vi "TSPopup.FG.Popup.vi"(4 "Popup Accepted?":bool, 6 "Popup Cluster Ref":refnum<vi>, 7 "Popup Operation":T5, 8 "error in (no error)":errorcluster, 9 "Font Size":u32, 10 "Encoded Location":string, 11 "Popup Parameters":T1) -> (0 "error out":errorcluster, 1 "Found":bool, 2 "Popup Parameters out":T1, 3 "Popup Event":refnum<user-event>)   [LabVIEW 2013]
doc: "The functional global that provides most of the functionality under the hood. This VI is wrapped by different public functions to provide a more user-friendly interface to the Type Sensitive Popup functions.\n\nType Sensitive Popup \nCopyright © 2007, J. David Saunders\nAll rights reserved."
uses:
  TSPopup.Popup Results.ctl
  TSPopup.Popup Operation.ctl
  TSPopup.Popup Call Parameters.ctl
  TSPopup.Data Type.ctl
  TSPopup.Monitor Register Data.ctl
  TSPopup.Event Enum.ctl
panel:
  in  "Reg. Data (type only)":T3
  in  "Popup Results (type only)":T6
  # "Type Sensitive Popup \nCopyright © 2007, J. David Saunders\nAll rights reserved."
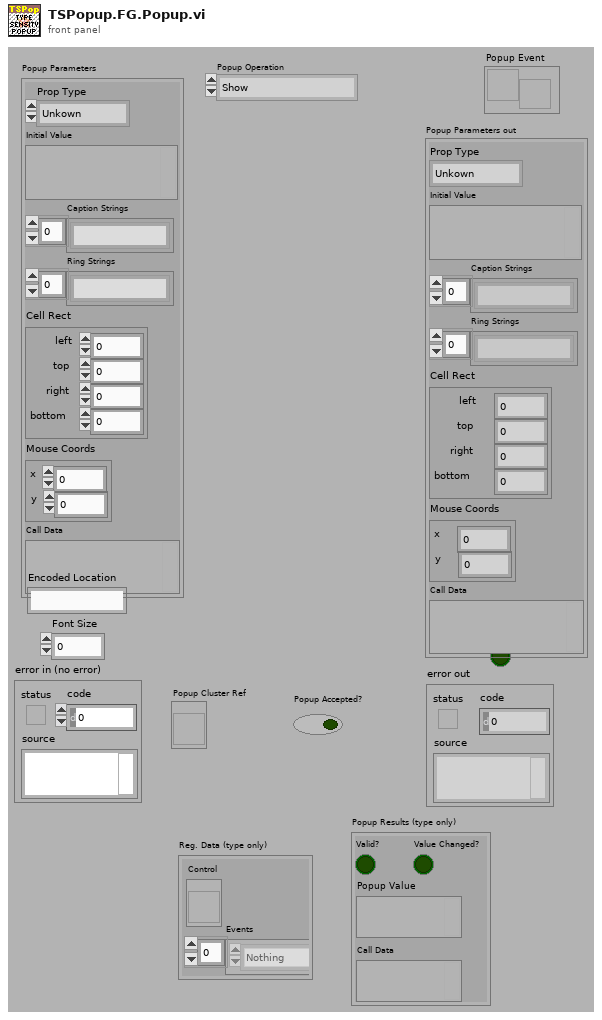
[diagram p1: front panel]
types:
  T1 = typedef "TSPopup.Popup Call Parameters.ctl" = cluster{"Prop Type":T2, "Initial Value":variant, "Caption Strings":string[], "Ring Strings":string[], "Cell Rect":cluster{"left":i16, "top":i16, "right":i16, "bottom":i16}, "Mouse Coords":cluster{"x":i16, "y":i16}, "Call Data":variant}
  T2 = typedef "TSPopup.Data Type.ctl" = enum16{"Unkown", "NO POPUP", "String", "Integer", "Float", "Color", "Boolean", "Ring", "Captioned String", "Captioned Integer", "Button Color", "2 Int Cluster", "4 Int Cluster"}
  T3 = typedef "TSPopup.Monitor Register Data.ctl" = cluster{"Control":refnum<vi>, "Events":T4[]}
  T4 = typedef "TSPopup.Event Enum.ctl" = enum16{"Nothing", "Enter Key Accept", "Escape Key Cancel", "Mouse Outside Accept", "Mouse Outside Cancel", "Mouse Move Accept", "Mouse Move Cancel", "Mouse Leave Cancel", "Value Change Accept", "Lose Focus Cancel", "Cancel Button", "Accept Button"}
  T5 = typedef "TSPopup.Popup Operation.ctl" = enum16{"Show", "Initialize", "Close", "Popup Done", "Register a Location's Type", "Retrieve Location's Type"}
  T6 = typedef "TSPopup.Popup Results.ctl" = cluster{"Valid?":bool, "Value Changed?":bool, "Popup Value":variant, "Call Data":variant}
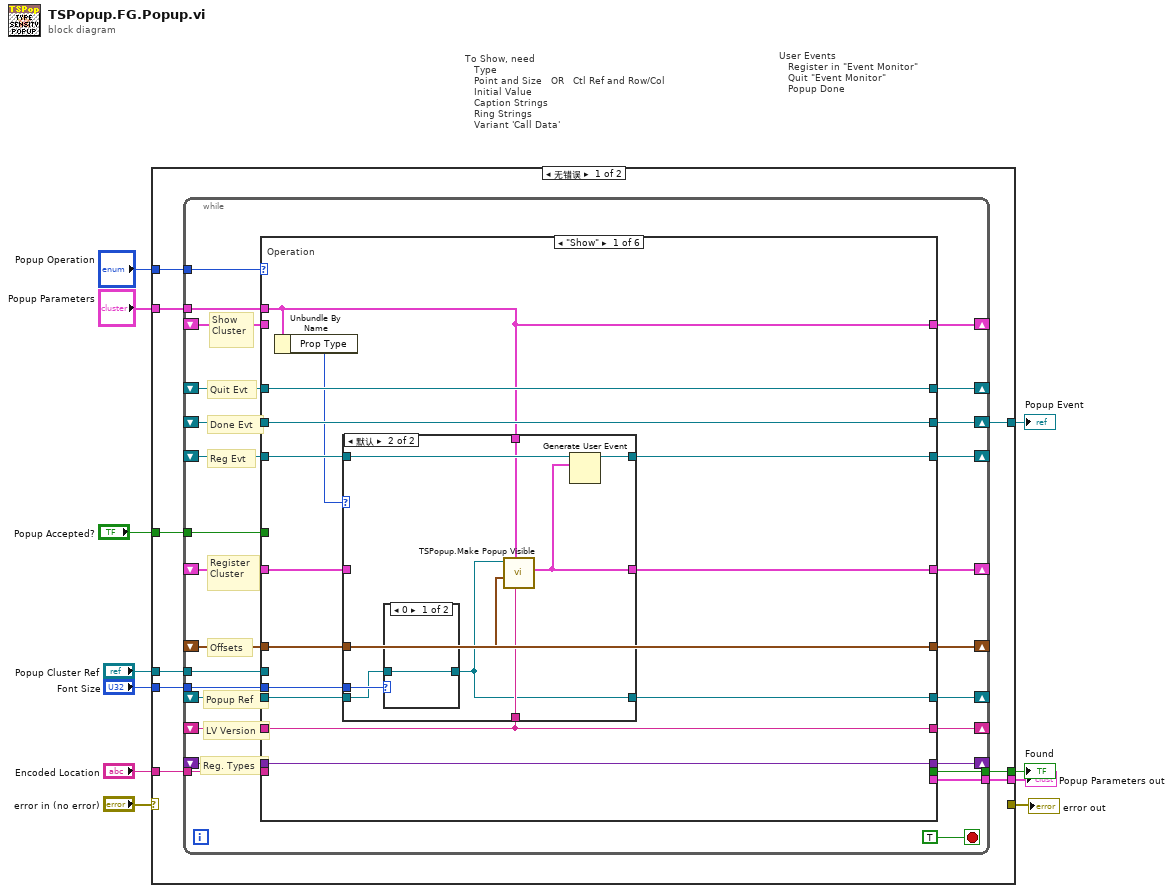
[diagram p0: block diagram]
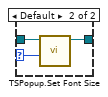
[diagram p3: hidden frame]
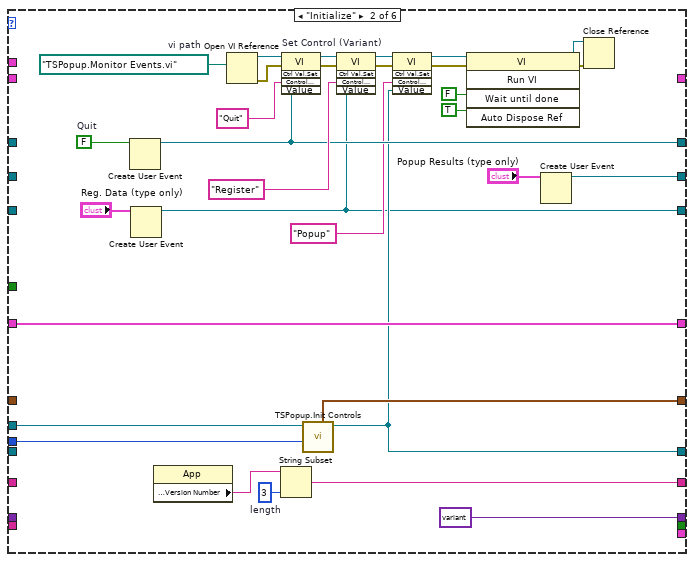
[diagram p4: hidden frame]
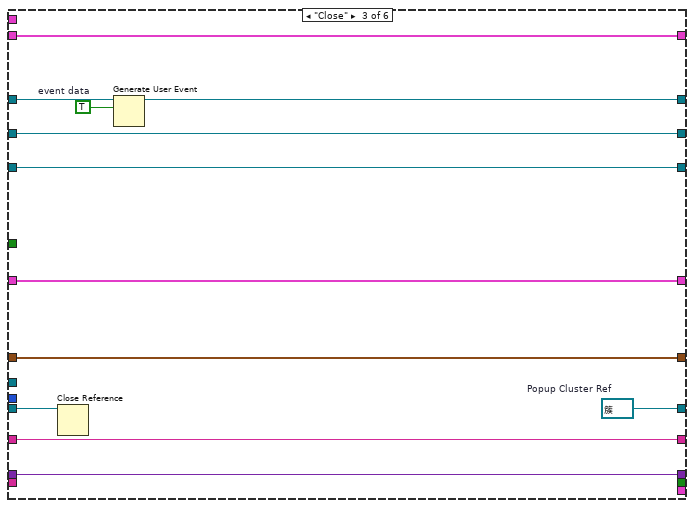
[diagram p5: hidden frame]
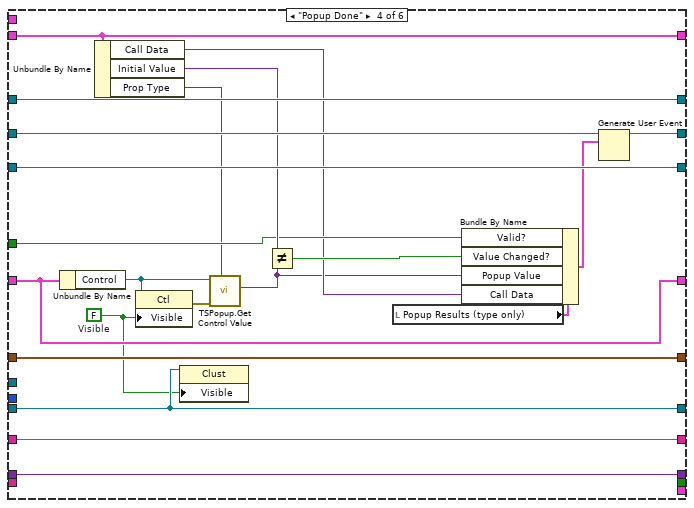
[diagram p6: hidden frame]
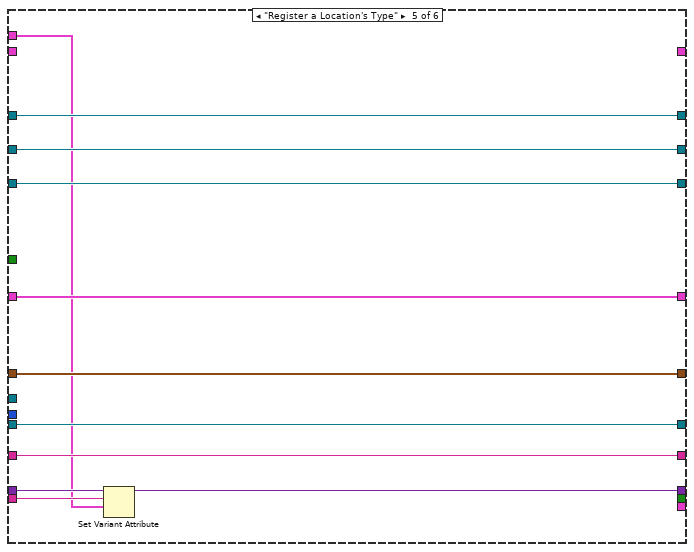
[diagram p7: hidden frame]
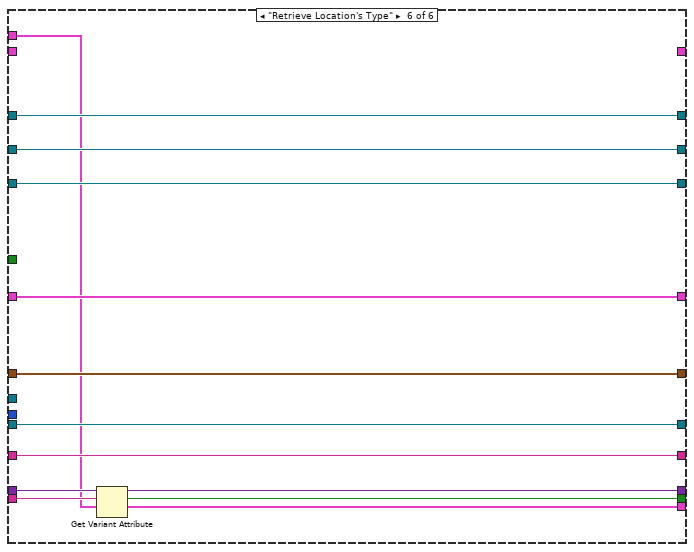
[diagram p8: hidden frame]
diagram:
  # "User Events\n   Register in \"Event Monitor\"\n   Quit \"Event Monitor\"\n   Popup Done"
  # "To Show, need\n   Type\n   Point and Size   OR   Ctl Ref and Row/Col\n   Initial Value\n   Caption Strings\n   Ring Strings\n   Variant 'Call Data'"
  n1 = case shown="无错误" "error in (no error)" {
    selector: "error in (no error)" -> [_ w166]
    tunnel: [_ w166] -> w11
    tunnel: "Popup Operation" -> [w20 _]
    tunnel: [w19 _] -> w8
    tunnel: "Popup Parameters" -> [w16 _]
    tunnel: "Popup Cluster Ref" -> [w18 _]
    tunnel: "Popup Accepted?" -> [w17 _]
    tunnel: "Encoded Location" -> [w15 _]
    tunnel: [w14 _] -> w3
    tunnel: [w13 _] -> w2
    tunnel: "Font Size" -> [w12 _]
    frame No Error {
      n2 = while {
        tunnel: w20 -> [w46]
        shift-right: [w45] -> _
        shift-left: _ -> [w44]
        shift-right: [w42] -> _
        shift-left: _ -> [w41]
        shift-right: [w43] -> w19
        shift-left: _ -> [w40]
        shift-right: [w38] -> _
        shift-left: _ -> [w39]
        shift-right: [w36] -> _
        shift-left: _ -> [w37]
        tunnel: w18 -> [w35]
        shift-right: [w34] -> _
        shift-left: _ -> [w33]
        shift-right: [w32] -> _
        shift-left: _ -> [w31]
        tunnel: w17 -> [w30]
        tunnel: w16 -> [w29]
        shift-right: [w28] -> _
        shift-left: _ -> [w27]
        shift-right: [w26] -> _
        shift-left: _ -> [w25]
        tunnel: w15 -> [w24]
        tunnel: [w23] -> w14
        tunnel: [w22] -> w13
        tunnel: w12 -> [w21]
        stop <- TRUE stop-if-true
        # "Reg. Types"
        # "LV Version"
        # "Popup Ref"
        # "Reg Evt"
        # "Done Evt"
        # "Quit Evt"
        # "Offsets"
        # "Register\nCluster"
        # "Show\nCluster"
        n3 = case "Operation" shown="\"Show\"" w46 {
          tunnel: [w61 w98 w118 w140 w152 w165] -> w45
          tunnel: w44 -> [w61 _ w120 w140 w152 w165]
          tunnel: [w60 w97 w116 w138 w151 w164] -> w43
          tunnel: [w48 w79 w117 w141 w150 w163] -> w42
          tunnel: w41 -> [w59 _ w117 w141 w150 w163]
          tunnel: w40 -> [w60 _ w116 w139 w151 w164]
          tunnel: w39 -> [_ _ w115 w137 _ _]
          tunnel: [w51 _ w115 w137 _ _] -> w38
          tunnel: [w52 w86 w111 w128 w147 w160] -> w36
          tunnel: w37 -> [w53 _ w112 w128 w147 w160]
          tunnel: w35 -> [_ w80 _ _ _ _]
          tunnel: [w58 w87 w114 w136 w148 w161] -> w34
          tunnel: w33 -> [w58 _ w114 w136 w148 w161]
          tunnel: [w57 w88 w113 w129 w149 w162] -> w32
          tunnel: w31 -> [w49 w88 w113 w129 w149 w162]
          tunnel: w30 -> [_ _ _ w131 _ _]
          tunnel: w29 -> [w51 _ _ _ w143 w156]
          tunnel: [w56 w83 w110 w122 w146 w159] -> w28
          tunnel: w27 -> [w56 _ w110 w122 w146 w159]
          tunnel: [w55 variant ("Variant") w109 w121 w142 w155] -> w26
          tunnel: w25 -> [w55 _ w109 w121 w145 w158]
          tunnel: w24 -> [_ _ _ _ w144 w157]
          tunnel: [_ _ _ _ _ w154] -> w23
          tunnel: [_ _ _ _ _ w153] -> w22
          tunnel: w21 -> [w54 w81 _ _ _ _]
          frame "Show" {
            n4 = Unbundle By Name(w51) -> ("Prop Type"=w50:T2)
            n5 = case shown="默认" w50 {
              tunnel: w59 -> [w64 w73]
              tunnel: [w64 w66] -> w48
              tunnel: w58 -> [_ w72]
              tunnel: [w63 w65] -> w57
              tunnel: w51 -> [_ w71]
              tunnel: w56 -> [_ w70]
              tunnel: w54 -> [_ w69]
              tunnel: w53 -> [w62 w68]
              tunnel: [w62 w67] -> w52
              tunnel: w49 -> [w63 _]
              frame "NO POPUP" {
              }
              frame Default {
                n6 = case shown="0" w69 {
                  selector: w69 -> [_ w77]
                  tunnel: w68 -> [w74 w76]
                  tunnel: [w74 w75] -> w67
                  frame 0 {
                  }
                  frame Default {
                    n7 = call "TSPopup.Set Font Size.vi"("Font Size"=w77, "Popup Cluster Ref"=w76) -> ("dup ref out"=w75:refnum<vi>)  [unwired: 8 in, 1 out]
                  }
                }
                n8 = call "TSPopup.Make Popup Visible.vi"("LV Version"=w70, "Popup Parameters"=w71, "Ctl Offsets"=w72, "Popup Cluster Ref"=w67) -> ("event data"=w65:T3)  [unwired: 6 in, 1 out]
                n9 = Generate User Event(user event=w73, event data cluster=w65) -> (user event out=w66:refnum<user-event>)  [unwired: 2 in, 1 out]
              }
            }
          }
          frame "Initialize" {
            w84 = 3  # length
            w78 = path "TSPopup.Monitor Events.vi"  # vi path
            w107 = FALSE  # Quit
            n10 = Create User Event(user event datatype=w107) -> (user event=w98:refnum<user-event>)  [unwired: 1 in, 1 out]
            n11 = Create User Event(user event datatype="Reg. Data (type only)") -> (user event=w79:refnum<user-event>)  [unwired: 1 in, 1 out]
            n12 = property class="App"() -> ("Application:Version Number"=w85:string)  [unwired: 2 in, 2 out]
            n13 = Open VI Reference(vi path=w78) -> (vi reference=w106:refnum<vi>, error out=w104:errorcluster)  [unwired: 5 in]
            n14 = String Subset(string=w85, length (rest)=w84) -> (substring=w83:string)  [unwired: 1 in]
            n15 = invoke on="Set Control (Variant)" class="VI" method="Ctrl Val.Set"(reference=w106, error in=w104, "Control Name"="Quit", "Value"=w98) -> (reference out=w95:refnum<vi>, error out=w96:errorcluster)  [unwired: 1 in, 3 out]
            n16 = call "TSPopup.Init Controls.vi"("Font Size"=w81, "Popup Cluster Ref"=w80) -> ("dup ref"=w86:refnum<vi>, "Offsets"=w87:cluster{"Left":i32, "Top":i32}[])  [unwired: 8 in]
            n17 = invoke on="Set Control (Variant)" class="VI" method="Ctrl Val.Set"(reference=w95, error in=w96, "Control Name"="Register", "Value"=w79) -> (reference out=w93:refnum<vi>, error out=w94:errorcluster)  [unwired: 1 in, 3 out]
            n18 = invoke on="Set Control (Variant)" class="VI" method="Ctrl Val.Set"(reference=w93, error in=w94, "Control Name"="Popup", "Value"=w86) -> (reference out=w92:refnum<vi>, error out=w91:errorcluster)  [unwired: 1 in, 3 out]
            n19 = invoke class="VI" method="Run VI"(reference=w92, error in=w91, "Wait until done"=FALSE, "Auto Dispose Ref"=TRUE ("Wait until done")) -> (reference out=w99:refnum<vi>, error out=w100:errorcluster)  [unwired: 1 in, 3 out]
            n20 = Create User Event(user event datatype="Popup Results (type only)") -> (user event=w97:refnum<user-event>)  [unwired: 1 in, 1 out]
            n21 = Close Reference(reference=w99, error in (no error)=w100) -> ()  [unwired: 1 out]
          }
          frame "Close" {
            w111 = refnum<vi> refnum  # Popup Cluster Ref
            w119 = TRUE  # event data
            n22 = Close Reference(reference=w112) -> ()  [unwired: 1 in, 1 out]
            n23 = Generate User Event(user event=w120, event data cluster=w119) -> (user event out=w118:refnum<user-event>)  [unwired: 2 in, 1 out]
          }
          frame "Popup Done" {
            w127 = FALSE  # Visible
            n24 = Unbundle By Name(w129) -> ("Control"=w126:refnum<vi>)
            n25 = Unbundle By Name(w137) -> ("Call Data"=w130:variant, "Initial Value"=w133:variant, "Prop Type"=w125:T2)
            n26 = property on="Property Node" class="Ctl"(reference=w126, "Visible"=w127) -> (error out=w123:errorcluster)  [unwired: 1 in, 1 out]
            n27 = property class="Clust"(reference=w128, "Visible"=w127) -> ()  [unwired: 1 in, 2 out]
            n28 = call "TSPopup.Get Control Value.vi"("Prop Type"=w125, "error in (no error)"=w123, "Control"=w126) -> ("Value"=w124:variant)  [unwired: 6 in, 2 out]
            n29 = Not Equal?(x=w133, y=w124) -> (x != y?=w132:bool)
            n30 = local read "Popup Results (type only)"() -> (w135:T6)
            n31 = Bundle By Name(cluster=w135, "Valid?"=w131, "Value Changed?"=w132, "Popup Value"=w124, "Call Data"=w130) -> (w134:T6)
            n32 = Generate User Event(user event=w139, event data cluster=w134) -> (user event out=w138:refnum<user-event>)  [unwired: 2 in, 1 out]
          }
          frame "Register a Location's Type" {
            n33 = Set Variant Attribute(Variant=w145, name=w144, value=w143) -> (Variant out=w142:variant)  [unwired: 1 in, 2 out]
          }
          frame "Retrieve Location's Type" {
            n34 = Get Variant Attribute(Variant=w158, name=w157, default value (empty Variant)=w156) -> (duplicate Variant=w155:variant, found=w154:bool, value=w153:T1)  [unwired: 1 in, 1 out]
          }
        }
      }
    }
    frame Error {
    }
  }
  "error out" <- w11
  "Popup Event" <- w8
  "Found" <- w3
  "Popup Parameters out" <- w2
